vi "SPECTOR_CoilConfigandFluxSelection.vi"(7 "Gun Flux":dbl(slide)=23.5 min=0.0 max=37.5 step=0.5 scale=0.0..40.0 scale format="%#_2g", 10 "Configuration":T1(ring)=enum."HUF - (High Upper Flux)") -> (0 "Max Gun Flux":dbl, 2 "Magnet Current Array":dbl[](array[numeric])=[0.0, 0.0, 127.0967741935484, 190.6451612903226, 67.741935483871] format="%#.1f", 3 "Magnets On":bool[](array[boolean]))   [LabVIEW 2016]
panel:
  in  "Gun Flux Values":dbl[][](array[numeric])=[[0.0, 9.0, 17.0, 24.0, 28.0, 31.0, 33.0, 35.0, 36.0], [0.0, 0.0, 0.0, 7.0, 13.0, 19.0, 22.3, 26.7, 29.0], [0.0, 0.0, 0.0, 16.1, 22.4, 25.5, 28.3, 30.6, 37.5]] caption="Gun Flux Lookup Values" format="%.1f"
  in  "CurrentLookup":i32[][][](array[numeric])=[[[0, 0, 0, 0, 0, 0, 0, 0, 0], [0, 0, 0, 0, 0, 0, 0, 0, 0], [0, 0, 0, 0, 0, 0, 0, 0, 0], [0, 0, 0, 0, 0, 0, 0, 0, 0], [0, 25, 50, 100, 200, 300, 400, 500, 600]], [[0, 0, 0, 0, 0, 0, 0, 0, 0], [0, 0, 0, 0, 0, 0, 0, 0, 0], [0, 0, 0, 0, 0, 0, 0, 0, 0], [0, 0, 0, 20, 39, 55, 68, 86, 100], [0, 0, 0, 25, 50, 75, 100, 200, 300]], [[0, 0, 0, 0, 0, 0, 0, 0, 0], [0, 0, 0, 0, 0, 0, 0, 0, 0], [0, 0, 0, 80, 120, 140, 180, 200, 300], [0, 0, 0, 120, 180, 210, 270, 300, 450], [0, 0, 0, 25, 50, 100, 200, 300, 600]]]
  # "This array gives the flux values (columns) as a function of configuration (rows) that correspond to the columns of coil currents \n\nTo determine flux values that do not fall on index values, linear interpolation will be used to get the intermediate value."
  # "Row"
  # "Col"
  # "Mag A"
  # "Page"
  # "This array is the lookup table of current values for the coils, for different \nflux amounts for the different coil configurations in SPECTOR\n\n    Row: A row correponds to a magnet (0..4 corresponds Mag A ... Mag E)\n    Col: Current value for the flux value in this column\n    Page: Configuration (MCO, LUF, HUF , etc ...)"
  # "Mag B"
  # "Row"
  # "Mag C (Upper Sand)"
  # "Col"
  # "Mag D (Lower Sand)"
  # "Mag E (Main Coil)"
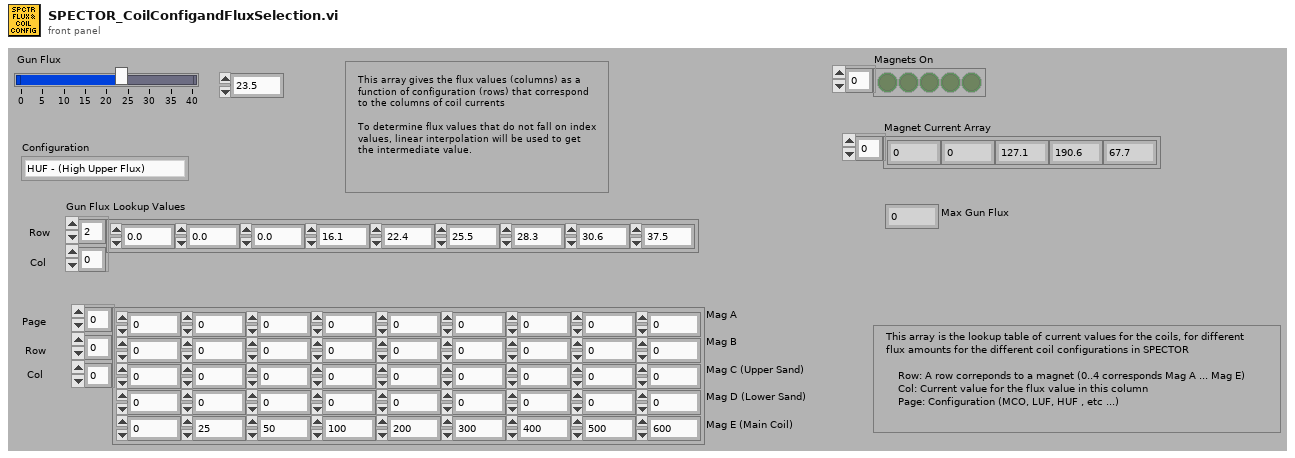
[diagram p1: front panel]
types:
  T1 = enum16{"MCO - (Main Coil Only)", "LUF - (Low Upper Flux)", "HUF - (High Upper Flux)"}
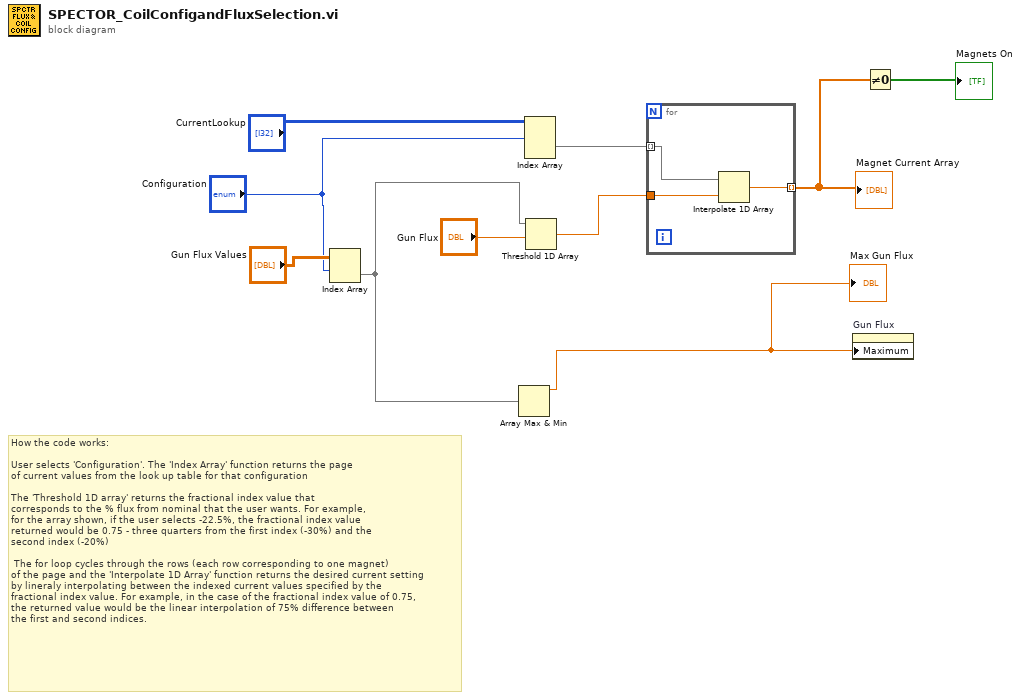
[diagram p0: block diagram]
diagram:
  # "How the code works:\n\nUser selects 'Configuration'. The 'Index Array' function returns the page \nof current values from the look up table for that configuration\n\nThe 'Threshold 1D array' returns the fractional index value that\ncorresponds to the % flux from nominal that the user wants. For example, \nfor the array shown, if the user selects -22.5%, the fractional index value \nreturned would be 0.75 - three quarters from the first index (-30%) and the\nsecond index (-20%)\n\n The for loop cycles through the rows (each row corresponding to one magnet) \nof the page and the 'Interpolate 1D Array' function returns the desired current setting \nby lineraly interpolating between the indexed current values specified by the  \nfractional index value. For example, in the case of the fractional index value of 0.75, \nthe returned value would be the linear interpolation of 75% difference between\nthe first and second indices."
  n1 = Index Array(array="Gun Flux Values", index (row)="Configuration") -> (element=w4:dbl[])  [unwired: 1 in]
  n2 = Array Max & Min(array=w4) -> (max value=w3:dbl)  [unwired: 3 out]
  "Max Gun Flux" <- w3
  n3 = Index Array(array="CurrentLookup", index (dim 0)="Configuration") -> (element=w8:i32[][])  [unwired: 2 in]
  n4 = Threshold 1D Array(2:"Gun Flux", 3:w4) -> (0:w7:dbl)  [unwired: 1 in]
  n5 = for {
    tunnel: w8 -> [w13] mode=indexing
    tunnel: w7 -> [w12]
    tunnel: [w11] -> w2 mode=indexing
    n6 = Interpolate 1D Array(1:w12, 2:w13) -> (0:w11:dbl)
  }
  "Magnet Current Array" <- w2
  n7 = property on="Gun Flux" class="Slide (strict)"("Maximum"=w3) -> ()  [unwired: 2 in, 2 out]
  n8 = Not Equal To 0?(x=w2) -> (x != 0?=→"Magnets On":bool[])
